vi "Get piezo voltage.vi"(0 "Piezo handle":i32, 11 "Piezo error in":errorcluster) -> (4 "Piezo handle out":i32, 6 "X Voltage":dbl, 8 "Y Voltage":dbl, 10 "Z Voltage":dbl, 15 "Piezo error out":errorcluster)   [LabVIEW 2017]
uses:
  <instrlib>/Thorlabs_MDT69xB/Thorlabs_MDT69xB.lvlib
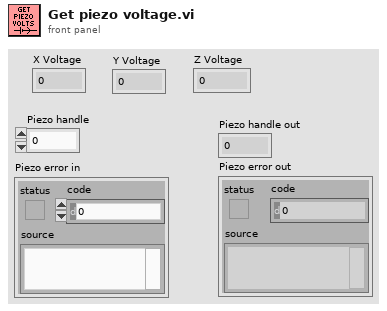
[diagram p1: front panel]
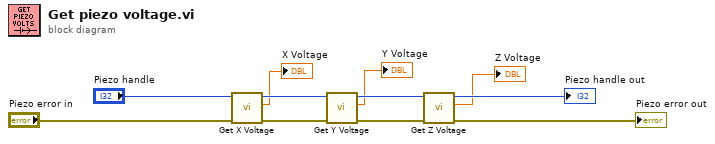
[diagram p0: block diagram]
diagram:
  n1 = call <instrlib>:"Get X Voltage.vi"("error in (no error)"="Piezo error in", "hdl in"="Piezo handle") -> ("error out"=w6:errorcluster, "x voltage"=→"X Voltage":dbl, "hdl"=w7:i32)  [unwired: 7 in]
  n2 = call <instrlib>:"Get Y Voltage.vi"("error in (no error)"=w6, "hdl in"=w7) -> ("error out"=w9:errorcluster, "y voltage"=→"Y Voltage":dbl, "hdl"=w8:i32)  [unwired: 7 in]
  n3 = call <instrlib>:"Get Z Voltage.vi"("error in (no error)"=w9, "hdl in"=w8) -> ("error out"=→"Piezo error out":errorcluster, "z voltage"=→"Z Voltage":dbl, "hdl"=→"Piezo handle out":i32)  [unwired: 7 in]
